vi "Post-Build Action Desktop.vi"(5 "Files Generated by Build":path[](array[path]), 6 "Top Level/Always Included VIs":path[](array[path]), 7 "Destination Path":path, 8 "error in (no error)":errorcluster, 9 "Target Name":string, 10 "Build Specification Name":string, 11 "Project Path":path) -> (0 "error out":errorcluster)   [LabVIEW 2017]
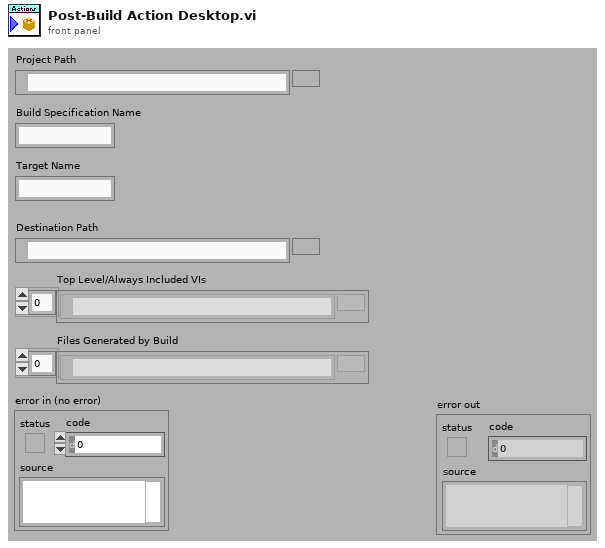
[diagram p1: front panel]
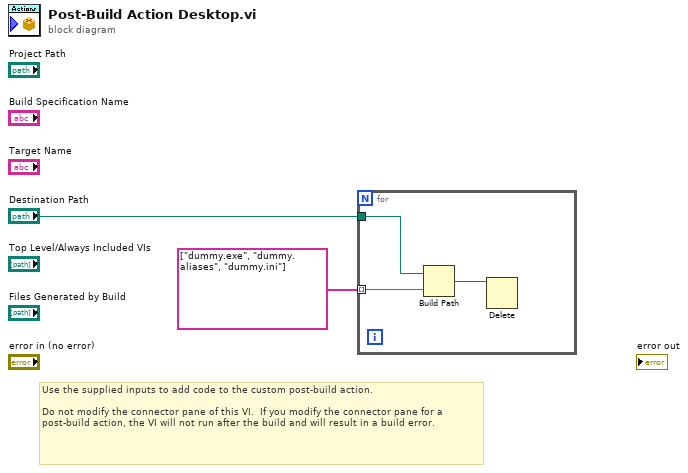
[diagram p0: block diagram]
diagram:
  # "Use the supplied inputs to add code to the custom post-build action.\n\nDo not modify the connector pane of this VI.  If you modify the connector pane for a post-build action, the VI will not run after the build and will result in a build error."
  n1 = for {
    tunnel: "Destination Path" -> [w5]
    tunnel: string[] ["dummy.exe", "dummy.aliases", "dummy.ini"] -> [w4] mode=indexing
    n2 = Build Path(base path=w5, name or relative path=w4) -> (appended path=w3:path)
    n3 = Delete(path (use dialog)=w3) -> ()  [unwired: 4 in, 3 out]
  }
